vi "Pick Up Order.vi"(8 "error in (no error)":errorcluster, 10 "Beverage":refnum<class "Beverage.lvclass">, 11 "Pick Up Order In":refnum<class "Pick Up Order.lvclass">) -> (0 "error out":errorcluster, 3 "Pick Up Order Out":refnum<class "Pick Up Order.lvclass">)   [LabVIEW 2020, in "Pick Up Order.lvclass"]
uses:
  Pick Up Order.lvclass
  Support/Beverages/Beverage/Beverage.lvclass
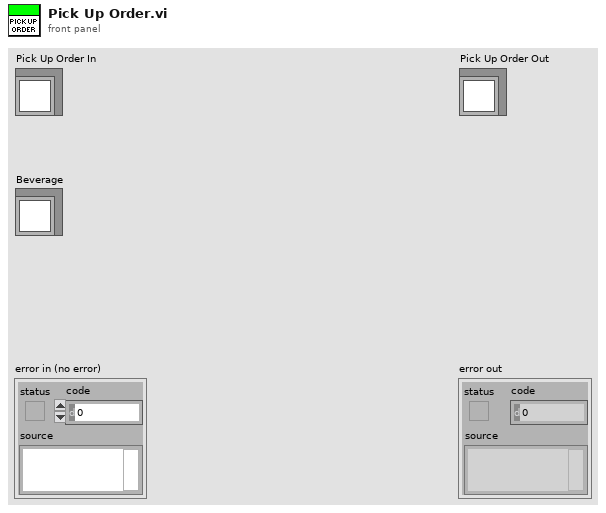
[diagram p1: front panel]
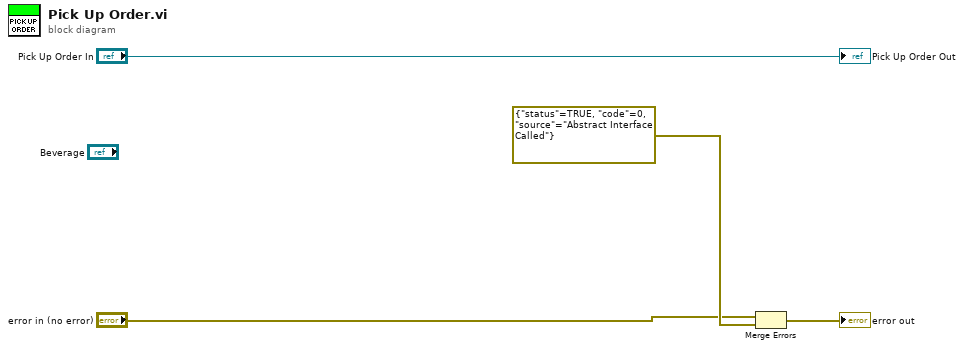
[diagram p0: block diagram]
diagram:
  n1 = Merge Errors("error in (no error)", errorcluster {"status"=TRUE, "code"=0, "source"="Abstract Interface Called"} ("error in (no error)")) -> (→"error out":errorcluster)
  "Pick Up Order Out" <- "Pick Up Order In"
